vi "GV FIFOIN timeout.vi"() -> ()   [LabVIEW 2017]
panel:
  out "FIFOINtimeout_tick":i32
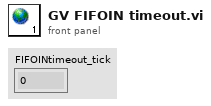
[diagram p1: front panel]
diagram:
